vi "distance_between_points_squared.vi"(3 "x LIDAR position":i16, 4 "y LIDAR position":i16, 5 "x position":i16, 6 "y position":i16) -> (1 "distance squared":i16)   [LabVIEW 2009]
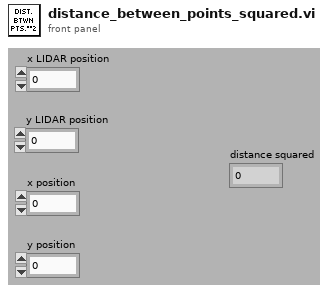
[diagram p1: front panel]
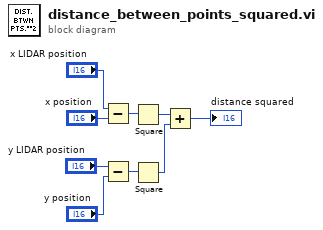
[diagram p0: block diagram]
diagram:
  n1 = Subtract(x="x LIDAR position", y="x position") -> (x-y=w6:i16)
  n2 = Subtract(x="y LIDAR position", y="y position") -> (x-y=w7:i16)
  n3 = Square(x=w6) -> (x^2=w9:i16)
  n4 = Square(x=w7) -> (x^2=w8:i16)
  n5 = Add(x=w9, y=w8) -> (x+y=→"distance squared":i16)
